vi "MHM Set Config.vi"(8 "error in (no error)":errorcluster, 9 "ulValue":u32, 10 "ulConfig":u32, 11 "ulMHMHandle":u32) -> (0 "error out":errorcluster, 3 "function return":u32)   [LabVIEW 2017, in "MHM_1SL_interface.lvlib"]
uses:
  MHM_1SL_interface.lvlib
  SSI_Tool/DUT_Interface/lv_interface/lib/MHM_1SL_interface.dll
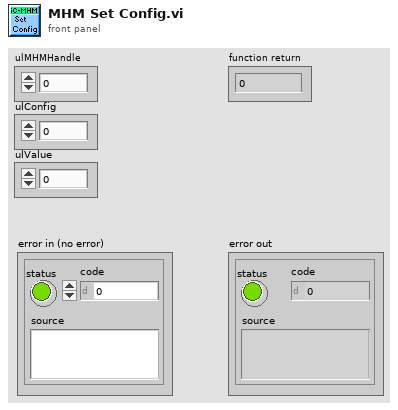
[diagram p1: front panel]
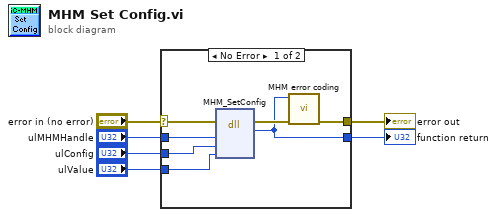
[diagram p0: block diagram]
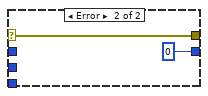
[diagram p2: hidden frame]
diagram:
  n1 = case shown="No Error" "error in (no error)" {
    selector: "error in (no error)" -> [w13 w15]
    tunnel: "ulMHMHandle" -> [w12 _]
    tunnel: "ulConfig" -> [w11 _]
    tunnel: "ulValue" -> [w10 _]
    tunnel: [w8 w15] -> w2
    tunnel: [w7 u32 0] -> w1
    frame No Error {
      n2 = dll-call lib="C:/workspace/project/scancon/sw/SSI_Tool/DUT_Interface/lv_interface/lib/MHM_1SL_interface.dll" fn="MHM_SetConfig"(error in=w13, "ulMHMHandle"=w12, "ulConfig"=w11, "ulValue"=w10) -> (error out=w9:errorcluster, "return type"=w7:u32)  [unwired: 5 in, 1 out]
      n3 = call "MHM error coding.vi"("error in (no error)"=w9, "function return in"=w7) -> ("error out"=w8:errorcluster)  [unwired: 9 in]
    }
    frame Error {
    }
  }
  "function return" <- w1
  "error out" <- w2
